vi "Help.vi"(5 "error in":errorcluster, 8 "TesterSWVersion":string) -> (0 "error out":errorcluster)   [LabVIEW 2017]
panel:
  out "String":string
  in  "Close":bool
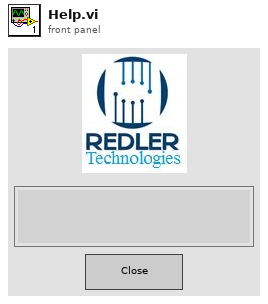
[diagram p1: front panel]
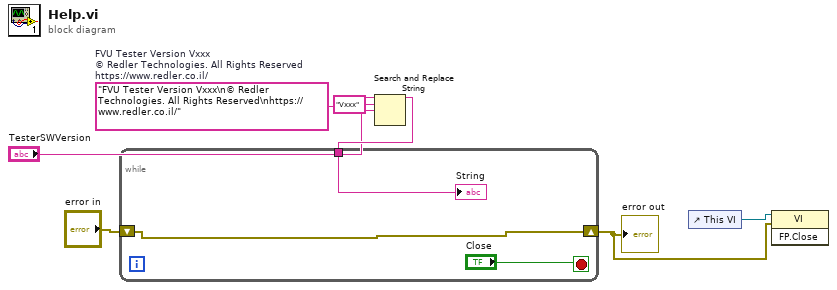
[diagram p0: block diagram]
diagram:
  w4 = "FVU Tester Version Vxxx\n© Redler Technologies. All Rights Reserved\nhttps://www.redler.co.il/"  # FVU Tester Version Vxxx © Redler Technologies. All Rights Reserved https://www.redler.co.il/
  n1 = Search and Replace String(input string=w4, search string="Vxxx", replace string="TesterSWVersion") -> (result string=w2:string)  [unwired: 5 in, 3 out]
  n2 = while {
    shift-right: [w9] -> w5
    shift-left: "error in" -> [w9]
    tunnel: w2 -> [w8]
    stop <- "Close" stop-if-true
    "String" <- w8
  }
  "error out" <- w5
  n3 = control-ref of="This VI"() -> (w6:refnum<vi>)
  n4 = invoke class="VI" method="FP.Close"(reference=w6, error in=w5) -> ()  [unwired: 1 in, 3 out]
